vi "ESP8266_Scan_IP.vi"() -> (3 "TCP Configuration":T1)   [LabVIEW 2018]
uses:
  <vilib>/MakerHub/LINX/Private/Device/Type Defs/TCP Config.ctl
  <vilib>/MakerHub/LINX/Public/Utilities/Open TCP.vi
  <vilib>/MakerHub/LINX/LMH-LINX.lvlib
  <vilib>/MakerHub/LINX/Private/Device/Device.lvlib
panel:
  out "status":bool
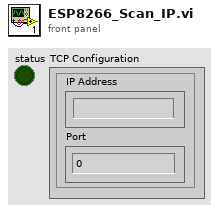
[diagram p1: front panel]
types:
  T1 = typedef "LMH-LINX.lvlib/Device.lvlib/TCP Config.ctl" = cluster{"IP Address":string, "Port":u16}
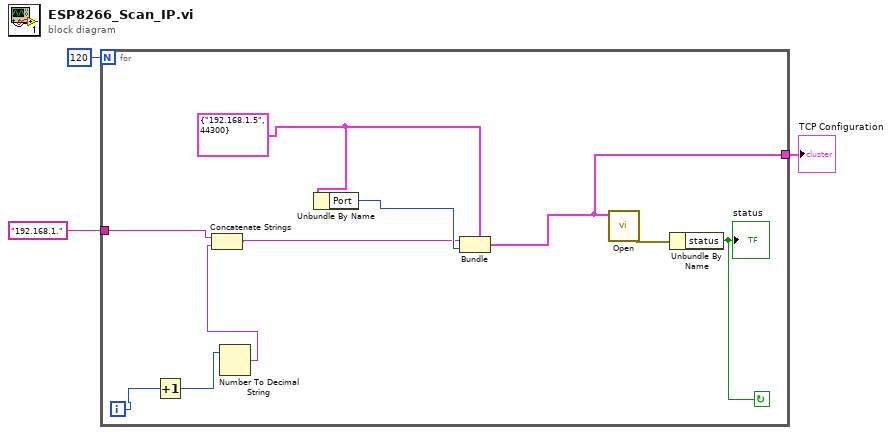
[diagram p0: block diagram]
diagram:
  n1 = for {
    N: 120 -> [_]
    tunnel: "192.168.1." ("IP Address") -> [w10]
    tunnel: [w4] -> w1
    i -> [w11]
    stop <- w5 continue-if-true
    w13 = T1 {"IP Address"="192.168.1.5", "Port"=44300} ("TCP Configuration")
    n2 = Increment(x=w11) -> (x+1=w8:i32)
    n3 = Number To Decimal String(number=w8) -> (decimal integer string=w7:string)  [unwired: 1 in]
    n4 = Concatenate Strings(w10, w7) -> (w9:string)
    n5 = Unbundle By Name(w13) -> ("Port"=w12:u16)
    n6 = Bundle(cluster=w13, "IP Address"=w9, "Port"=w12) -> (w4:T1)
    n7 = call-poly <vilib>:"Open.vi"("TCP Configuration"=w4) -> ("Error Out"=w6:errorcluster)  [unwired: 8 in, 2 out]
    n8 = Unbundle By Name(w6) -> ("status"=w5:bool)
    "status" <- w5
  }
  "TCP Configuration" <- w1
